vi "Test GPIB.vi"() -> ()   [LabVIEW 2015]
uses:
  <vilib>/Platform/TimedLoop/XDataNode/timing_clust.ctl
  <vilib>/Platform/TimedLoop/XDataNode/nitl_modes.ctl
  <vilib>/Platform/TimedLoop/XDataNode/wakeup.ctl
  <vilib>/platform/TimedLoop/XDataNode/XDataNode.xnode
  <vilib>/Platform/TimedLoop/XDataNode/XDNodeRunTimeDep.lvlib
panel:
  out "Cmd Str":string
  out "error out":errorcluster
  in  "Stop Button":bool
  out "read buffer":string
  in  "VISA resource name":refnum<visa-resource-name>
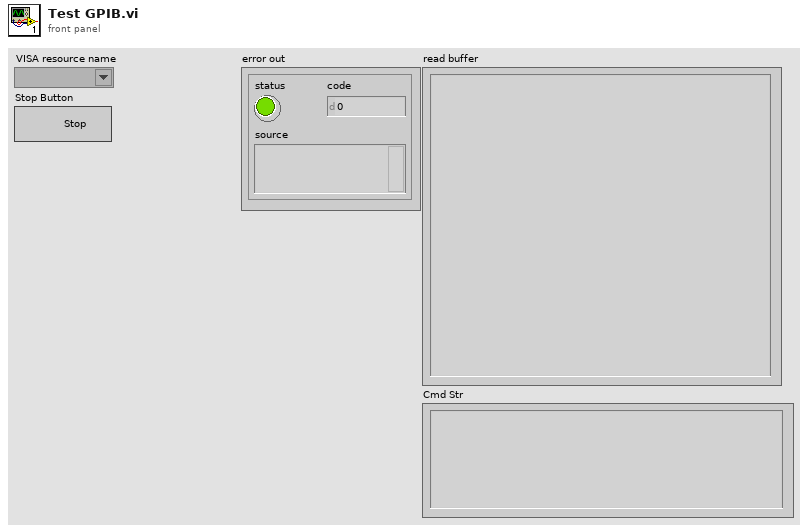
[diagram p1: front panel]
types:
  T1 = typedef "XDNodeRunTimeDep.lvlib/timing_clust.ctl" = cluster{"Expected End [f-1]":u64, "Actual End [f-1]":u64, "Finished Late? [f-1]":bool, "Expected End [i-1]":u64, "Actual End [i-1]":u64, "Finished Late? [i-1]":bool, "Expected Start [i]":u64, "Actual Start [i]":u64, "Expected Start [f]":u64, "Actual Start [f]":u64, "Source Name":string, "Structure Name":string, "Period":i64, "Deadline":i64, "Offset":i64, "Start":i64, "Priority":i32, "Timeout":i32, "Mode":T2, "Wakeup Reason":T3, "Error":errorcluster, "Source Type":string, "Secondary Source Type":string, "Global End Time":u64, "Global Start Time":u64, "Frame Duration":u64, "Iteration Duration":u64, "Assigned CPU":i32, "I/O Scan Engine Mode":u32}
  T2 = typedef "XDNodeRunTimeDep.lvlib/nitl_modes.ctl" = enum32{"No Change", "Process missed periods, maintain original phase", "Discard missed periods, maintain original phase", "Process missed periods, ignore original phase", "Discard missed periods, ignore original phase"}
  T3 = typedef "XDNodeRunTimeDep.lvlib/wakeup.ctl" = enum32{"Normal", "Aborted", "Asynchronous wakeup", "Timing source error", "Timed loop error", "Timeout"}
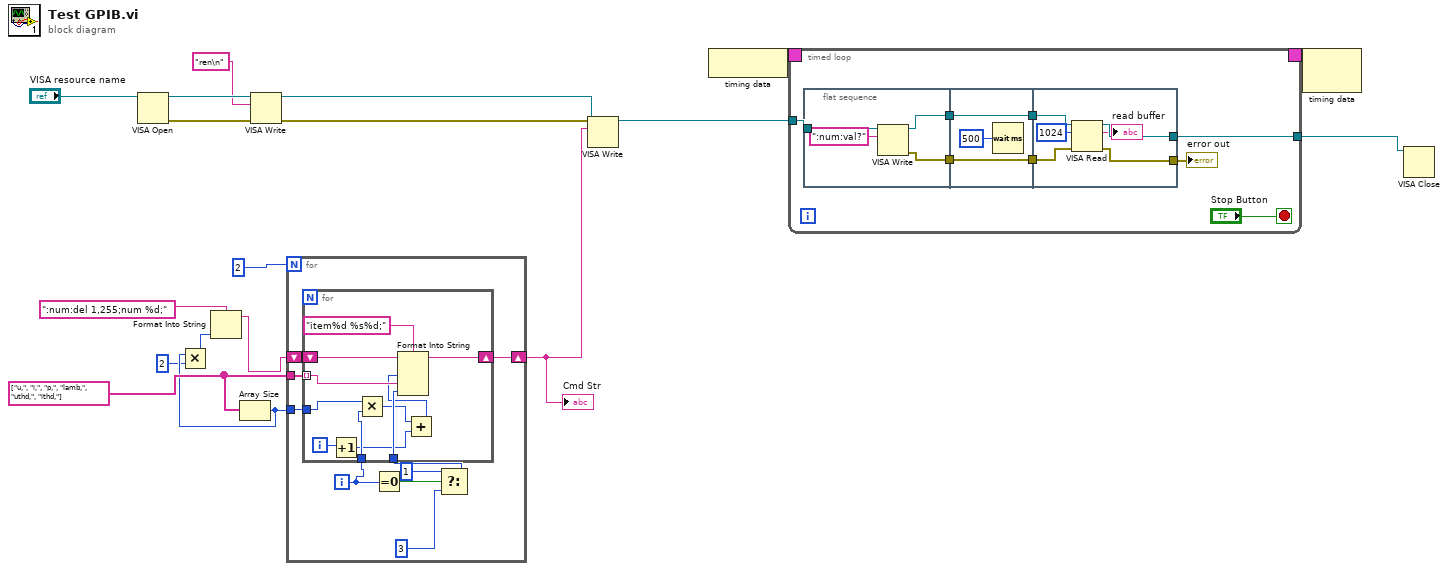
[diagram p0: block diagram]
diagram:
  w6 = string[] ["u,", "i,", "p,", "lamb,", "uthd,", "ithd,"]
  n1 = VISA Open(VISA resource name="VISA resource name") -> (VISA resource name=w17:refnum<visa-resource-name>, error out=w16:errorcluster)  [unwired: 4 in]
  n2 = Array Size(array=w6) -> (size(s)=w3:i32)
  n3 = Multiply(x=w3, y=2) -> (x*y=w1:i32)
  n4 = Format Into String(format string=":num:del 1,255;num %d;", w1) -> (resulting string=w4:string)  [unwired: 2 in, 1 out]
  n5 = VISA Write(VISA resource name=w17, write buffer="ren\n", error in (no error)=w16) -> (VISA resource name out=w14:refnum<visa-resource-name>, error out=w13:errorcluster)  [unwired: 1 out]
  n6 = for {
    N: 2 -> [_]
    shift-right: [w25] -> w7
    shift-left: w4 -> [w27]
    tunnel: w6 -> [w26]
    tunnel: w3 -> [w24]
    i -> [w23]
    n7 = Equal To 0?(x=w23) -> (x = 0?=w22:bool)
    n8 = Select(t=1, s=w22, f=3) -> (s? t:f=w19:i32)
    n9 = for {
      shift-right: [w36] -> w25
      shift-left: w27 -> [w37]
      tunnel: w26 -> [w35] mode=indexing
      tunnel: w19 -> [w33]
      tunnel: w23 -> [w31]
      tunnel: w24 -> [w32]
      i -> [w34]
      n10 = Increment(x=w34) -> (x+1=w29:i32)
      n11 = Multiply(x=w32, y=w31) -> (x*y=w30:i32)
      n12 = Add(x=w30, y=w29) -> (x+y=w28:i32)
      n13 = Format Into String(format string="item%d %s%d;", initial string=w37, w28, w35, w33) -> (resulting string=w36:string)  [unwired: 1 in, 1 out]
    }
  }
  "Cmd Str" <- w7
  n14 = VISA Write(VISA resource name=w14, write buffer=w7, error in (no error)=w13) -> (VISA resource name out=w10:refnum<visa-resource-name>)  [unwired: 2 out]
  n15 = node-c288() -> (w12:T1)
  n16 = timed-loop {
    timing: w12 -> [_]
    timing-out: [_] -> w11
    tunnel: w10 -> [w45]
    tunnel: [w42] -> w9
    stop <- "Stop Button" stop-if-true
    n17 = flat-sequence {
      tunnel: w45 -> [w50]
      tunnel: [w48] -> w43
      tunnel: [w47] -> w40
      tunnel: [w52] -> w44
      tunnel: w43 -> [w52]
      tunnel: [w51] -> w41
      tunnel: w40 -> [w51]
      tunnel: [w58] -> w42
      tunnel: [w57] -> w39
      tunnel: w44 -> [w55]
      tunnel: w41 -> [w54]
      frame #0 {
        n18 = VISA Write(VISA resource name=w50, write buffer=":num:val?") -> (VISA resource name out=w48:refnum<visa-resource-name>, error out=w47:errorcluster)  [unwired: 1 in, 1 out]
      }
      frame #1 {
        n19 = Wait (ms)(milliseconds to wait=u32 500) -> ()  [unwired: 1 out]
      }
      frame #2 {
        n20 = VISA Read(VISA resource name=w55, byte count=u32 1024, error in (no error)=w54) -> (VISA resource name out=w58:refnum<visa-resource-name>, read buffer=→"read buffer":string, error out=w57:errorcluster)  [unwired: 1 out]
      }
    }
    "error out" <- w39
  }
  n21 = node-c288(w11) -> ()  [unwired: 1 out]
  n22 = VISA Close(VISA resource name=w9) -> ()  [unwired: 1 in, 1 out]
